vi "MaeanderDemo.vi"(0 "lLSID":i32, 1 "Maeander Parameter":T1={"Number"=5, "X Start"=0.0, "Y Start"=0.0, "X Size"=2.0, "Y Size"=20.0} {"Y Size" format="%.6f"; "X Size" format="%.6f"; "Y Start" format="%.6f"; "X Start" format="%.6f"}, 3 "error in (no error)":errorcluster) -> (9 "error out":errorcluster)   [LabVIEW 2011]
uses:
  Maeander_Param.ctl
  <userlib>/Tango_DLL/Tango_DLL.lvlib
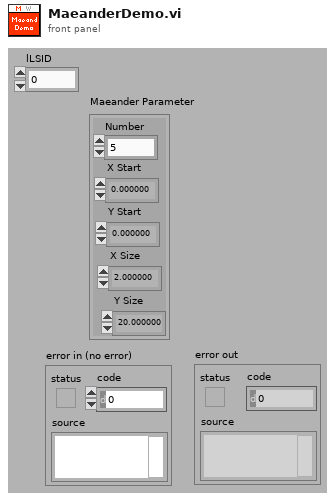
[diagram p1: front panel]
types:
  T1 = typedef "Maeander_Param.ctl" = cluster{"Number":i32, "X Start":dbl, "Y Start":dbl, "X Size":dbl, "Y Size":dbl}
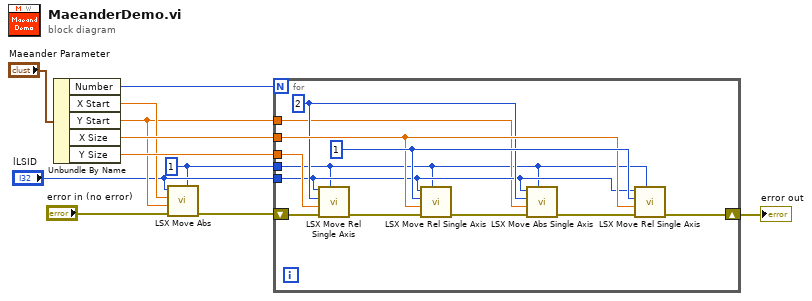
[diagram p0: block diagram]
diagram:
  w1 = 1 ("bWait")
  n1 = Unbundle By Name("Maeander Parameter") -> ("Number"=w10:i32, "X Start"=w6:dbl, "Y Start"=w5:dbl, "X Size"=w9:dbl, "Y Size"=w8:dbl)
  n2 = call <userlib>:"LSX Move Abs.vi"("bWait"=w1, "error in (no error)"="error in (no error)", "dY"=w5, "dX"=w6, "lLSID"="lLSID") -> ("error out"=w2:errorcluster)  [unwired: 5 in, 1 out]
  n3 = for {
    N: w10 -> [_]
    shift-right: [w13] -> w11
    shift-left: w2 -> [w23]
    tunnel: w5 -> [w17]
    tunnel: w9 -> [w20]
    tunnel: w8 -> [w22]
    tunnel: "lLSID" -> [w18]
    tunnel: w1 -> [w12]
    w19 = 2 ("lAxis")
    w21 = 1 ("lAxis")
    n4 = call <userlib>:"LSX Move Rel Single Axis.vi"("bWait"=w12, "error in (no error)"=w23, "dValue"=w22, "lAxis"=w19, "lLSID"=w18) -> ("error out"=w16:errorcluster)  [unwired: 5 in, 1 out]
    n5 = call <userlib>:"LSX Move Rel Single Axis.vi"("bWait"=w12, "error in (no error)"=w16, "dValue"=w20, "lAxis"=w21, "lLSID"=w18) -> ("error out"=w15:errorcluster)  [unwired: 5 in, 1 out]
    n6 = call <userlib>:"LSX Move Abs Single Axis.vi"("bWait"=w12, "error in (no error)"=w15, "dValue"=w17, "lAxis"=w19, "lLSID"=w18) -> ("error out"=w14:errorcluster)  [unwired: 5 in, 1 out]
    n7 = call <userlib>:"LSX Move Rel Single Axis.vi"("bWait"=w12, "error in (no error)"=w14, "dValue"=w20, "lAxis"=w21, "lLSID"=w18) -> ("error out"=w13:errorcluster)  [unwired: 5 in, 1 out]
  }
  "error out" <- w11
